vi "Настройки мишени (Sub VI).vi"(2 "Параметры мишеней вх":T1, 5 "error in":errorcluster) -> (16 "Параметры мишеней вых":T1, 19 "error out":errorcluster)   [LabVIEW 2013]
doc: "Подпрограмма управления мишенями: создание новой мишени и редактирование существующих"
panel:
  in  "Настройки мишени:":string
  in  "Ширина, мм":u16
  in  "Длина, мм":u16
  in  "Шаг перехода по вертикали":dbl min=0.0 format="%.1f"
  in  "Шаг перехода по горизонтали":dbl min=0.0 format="%.1f"
  in  "Выстрелов до перехода":u16
  in  "Отмена":bool
  in  "Y0":u16
  in  "Х0":u16
  in  "Сохранить настройки":bool
  # "Положение:"
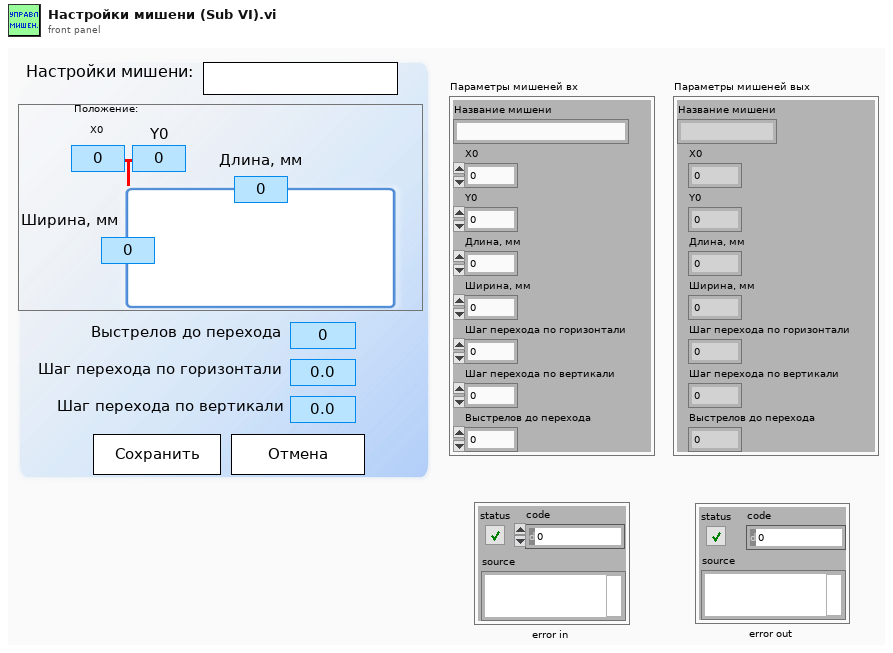
[diagram p1: front panel]
types:
  T1 = cluster{"Название мишени":string, "Х0":u16, "Y0":u16, "Длина, мм":u16, "Ширина, мм":u16, "Шаг перехода по горизонтали":u16, "Шаг перехода по вертикали":u16, "Выстрелов до перехода":u16}
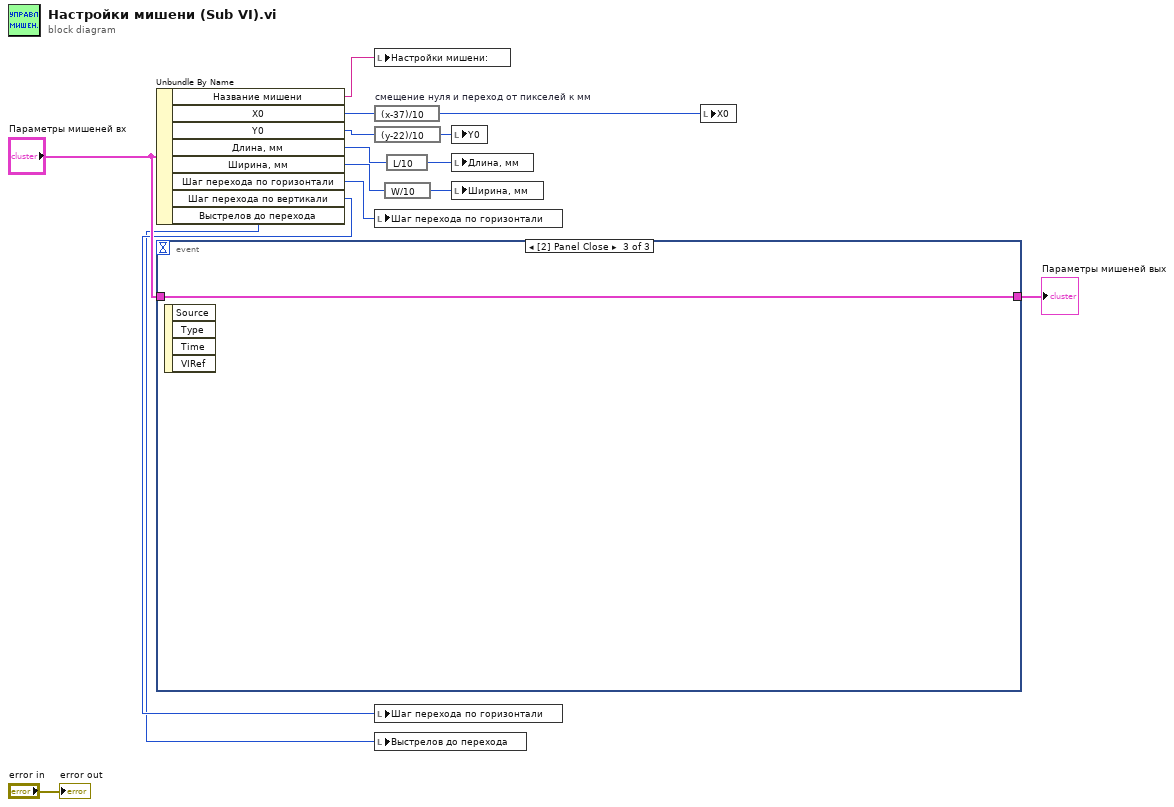
[diagram p0: block diagram]
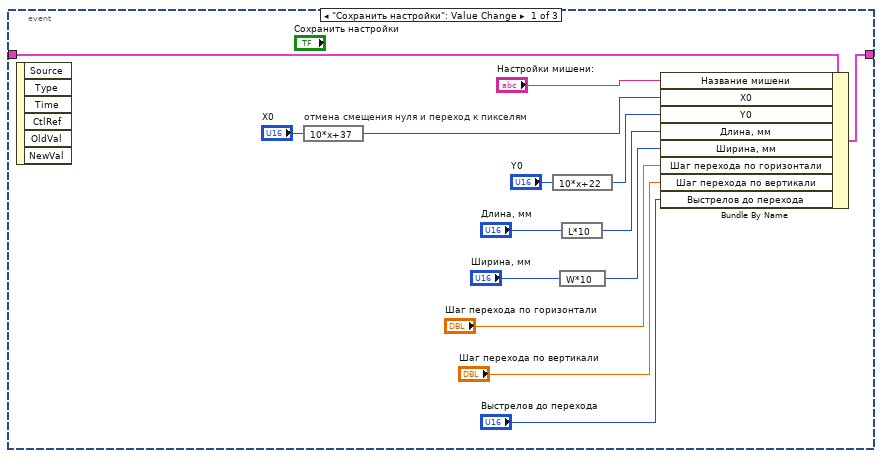
[diagram p2: hidden frame]
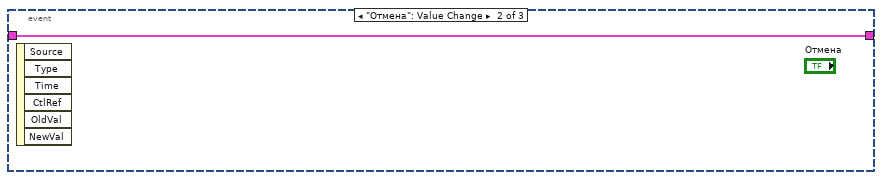
[diagram p3: hidden frame]
diagram:
  n1 = Unbundle By Name("Параметры мишеней вх") -> ("Название мишени"=w12:string, "Х0"=w8:u16, "Y0"=w7:u16, "Длина, мм"=w4:u16, "Ширина, мм"=w2:u16, "Шаг перехода по горизонтали"=w11:u16, "Шаг перехода по вертикали"=w10:u16, "Выстрелов до перехода"=w9:u16)
  n2 = event shown="[2] Panel Close" {
    selector: _ -> [_ _ _]
    dyn-events: _ -> [_ _ _]
    timeout: _ -> [_ _ _]
    tunnel: [w29 w30 w31] -> w14
    tunnel: "Параметры мишеней вх" -> [w28 w30 w31]
    event "Сохранить настройки": Value Change {
      n3 = event-data() -> ()  [unwired: 1 in, 6 out]
      n4 = expression code="10*x+37" "отмена смещения нуля и переход к пикселям"("Х0") -> (w22:u16)
      n5 = expression code="10*x+22"("Y0") -> (w21:u16)
      n6 = expression code="W*10"("Ширина, мм") -> (w17:u16)
      n7 = expression code="L*10"("Длина, мм") -> (w19:u16)
      n8 = Bundle By Name(cluster=w28, "Название мишени"="Настройки мишени:", "Х0"=w22, "Y0"=w21, "Длина, мм"=w19, "Ширина, мм"=w17, "Шаг перехода по горизонтали"="Шаг перехода по горизонтали", "Шаг перехода по вертикали"="Шаг перехода по вертикали", "Выстрелов до перехода"="Выстрелов до перехода") -> (w29:T1)
    }
    event "Отмена": Value Change {
      n9 = event-data() -> ()  [unwired: 1 in, 6 out]
    }
    event Panel Close {
      n10 = event-data() -> ()  [unwired: 1 in, 4 out]
    }
  }
  "Параметры мишеней вых" <- w14
  n11 = local write "Настройки мишени:"(w12) -> ()
  n12 = expression code="(x-37)/10" "смещение нуля и переход от пикселей к мм"(w8) -> (w6:u16)
  n13 = expression code="(y-22)/10"(w7) -> (w5:u16)
  n14 = local write "Шаг перехода по горизонтали"(w11) -> ()
  n15 = local write "Шаг перехода по горизонтали"(w10) -> ()
  n16 = local write "Выстрелов до перехода"(w9) -> ()
  n17 = expression code="W/10"(w2) -> (w1:u16)
  n18 = expression code="L/10"(w4) -> (w3:u16)
  n19 = local write "Y0"(w5) -> ()
  n20 = local write "Длина, мм"(w3) -> ()
  n21 = local write "Ширина, мм"(w1) -> ()
  n22 = local write "Х0"(w6) -> ()
  "error out" <- "error in"
